vi "MicrometerDryRun.vi"() -> ()   [LabVIEW 2015]
uses:
  <vilib>/Analysis/baseanly.llb/Mean (DBL).vi
  <vilib>/Analysis/NI_AALBase.lvlib
panel:
  in  "Done ?":bool
  out "nome file":string="micrometer_"
  in  "suffisso (se necessario)":string
  out "rms value":dbl format="%0.2f"
  out "mean":dbl format="%0.2f"
  out "appended array":dbl[](array[numeric])
  in  "stop":bool
  in  "2200,500":dbl format="%.2g"
  in  "0,500":dbl format="%.2g"
  in  "0,400":dbl format="%.2g"
  in  "2000,200":dbl format="%.2g"
  in  "1550,200":dbl format="%.2g"
  in  "1200,200":dbl format="%.2g"
  in  "800,200":dbl format="%.2g"
  in  "200,200":dbl format="%.2g"
  in  "2000,1100":dbl format="%.2g"
  in  "1550,1100":dbl format="%.2g"
  in  "1200, 1100":dbl format="%.2g"
  in  "800,1100":dbl format="%.2g"
  in  "200,1100":dbl format="%.2g"
  # "Dry Run"
  # "- Scrivi i valori delle misure effettuate con il micrometro nelle                                  caselle corrispondenti\n- Aggiungi il suffisso al nome del file (se necessario)\n- clicca su \"DONE\" quando hai immesso tutti i valori"
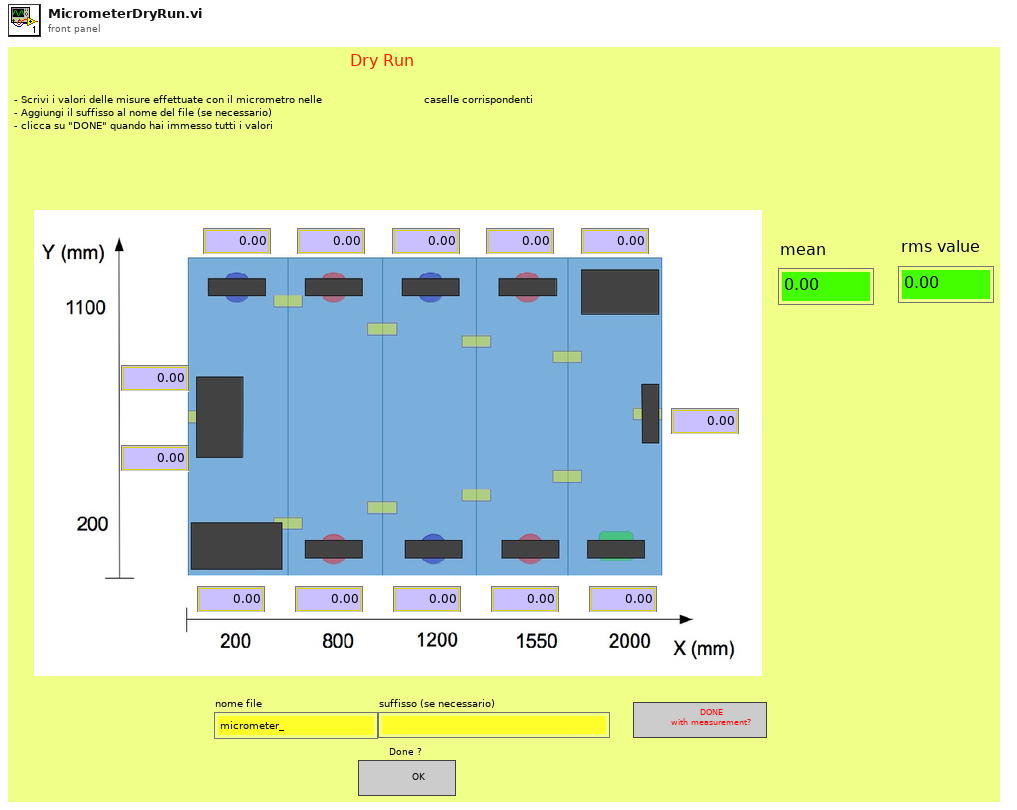
[diagram p1: front panel]
types:
  T1 = enum16{"open", "replace", "create", "open or create", "replace or create", "replace or create with confirmation"}
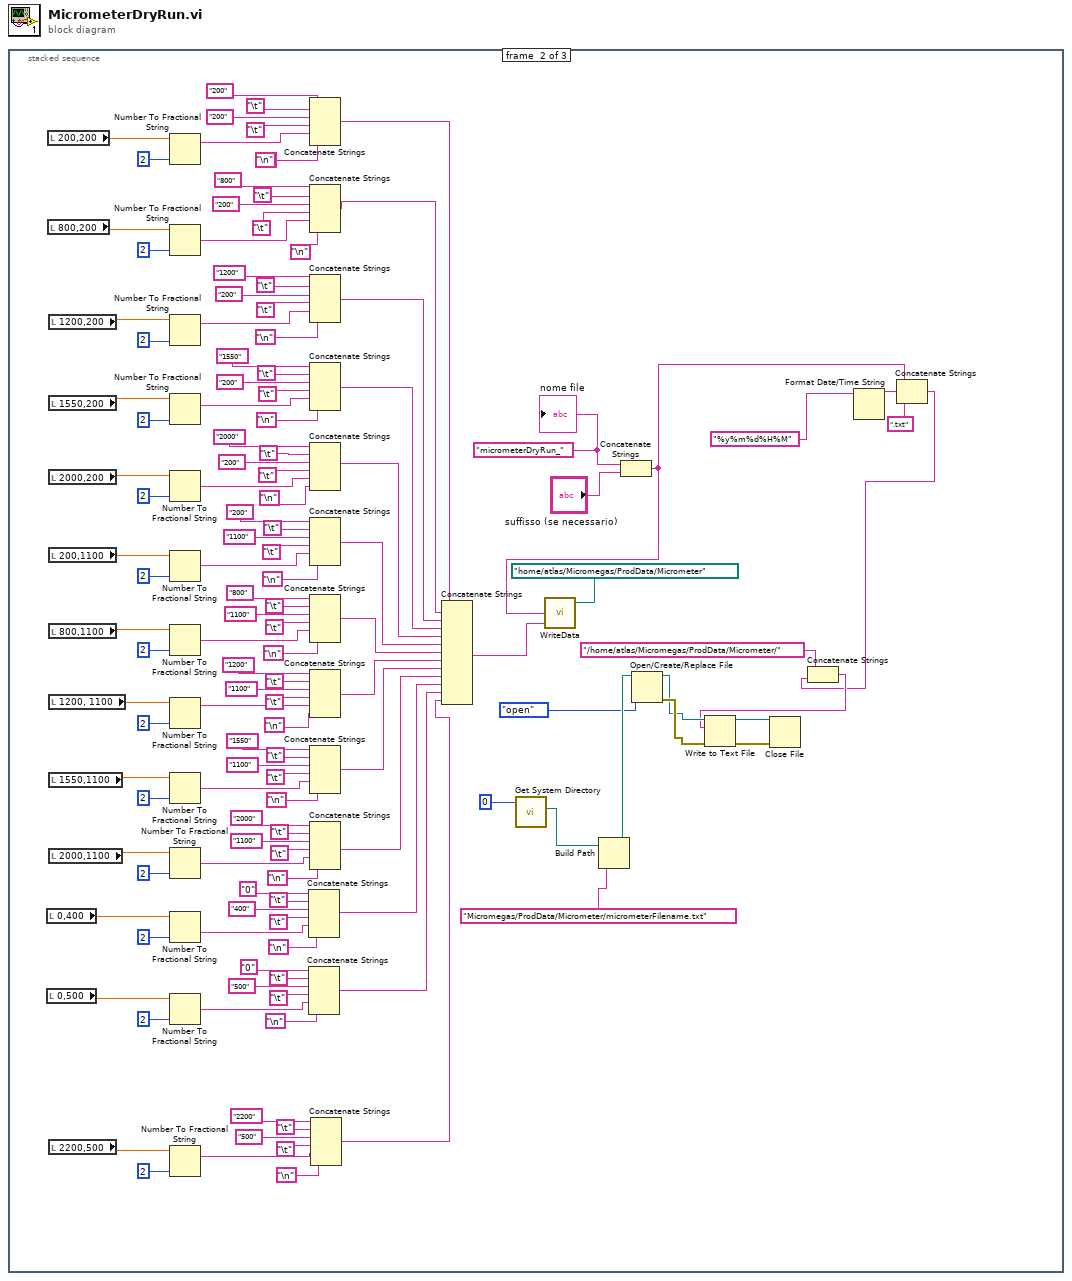
[diagram p0: block diagram]
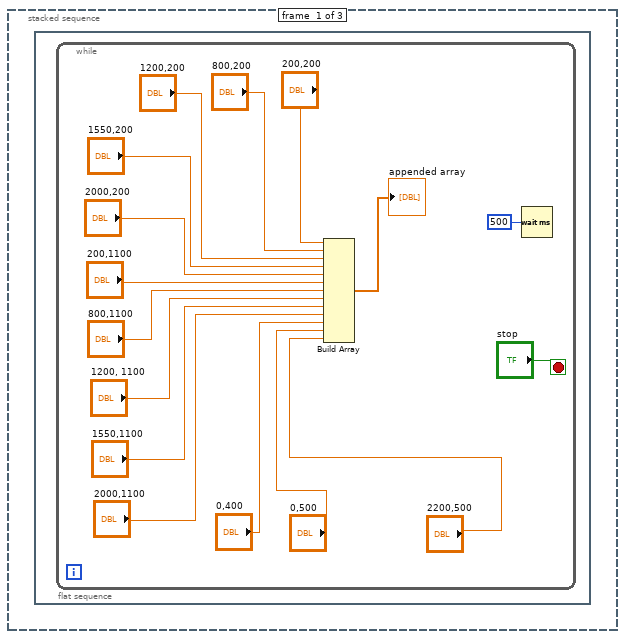
[diagram p2: hidden frame]
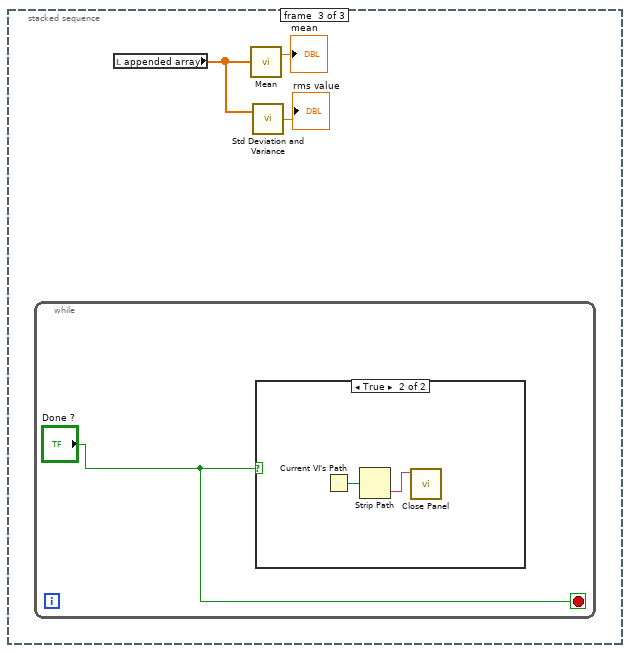
[diagram p3: hidden frame]
diagram:
  n1 = stacked-sequence {
    frame #0 {
      n2 = flat-sequence {
        frame #0 {
          n3 = while {
            stop <- "stop" stop-if-true
            n4 = Build Array("200,200", "800,200", "1200,200", "1550,200", "2000,200", "200,1100", "800,1100", "1200, 1100", "1550,1100", "2000,1100", "0,400", "0,500", "2200,500") -> (→"appended array":dbl[])
            n5 = Wait (ms)(milliseconds to wait=u32 500) -> ()  [unwired: 1 out]
          }
        }
      }
    }
    frame #1 {
      w36 = "micrometerDryRun_" ("string")
      (unwired) "\n"
      n6 = local read "0,400"() -> (w56:dbl)
      n7 = local read "0,500"() -> (w55:dbl)
      n8 = local read "200,200"() -> (w139:dbl)
      n9 = local read "800,200"() -> (w138:dbl)
      n10 = local read "1200,200"() -> (w116:dbl)
      n11 = local read "1550,200"() -> (w115:dbl)
      n12 = local read "2000,200"() -> (w114:dbl)
      n13 = local read "200,1100"() -> (w79:dbl)
      n14 = local read "800,1100"() -> (w78:dbl)
      n15 = local read "1200, 1100"() -> (w77:dbl)
      n16 = local read "1550,1100"() -> (w76:dbl)
      n17 = local read "2000,1100"() -> (w75:dbl)
      n18 = local read "2200,500"() -> (w54:dbl)
      n19 = Number To Fractional String(number=w139, precision (6)=i16 2) -> (F-format string=w148:string)  [unwired: 2 in]
      n20 = Number To Fractional String(number=w138, precision (6)=i16 2) -> (F-format string=w142:string)  [unwired: 2 in]
      n21 = Number To Fractional String(number=w116, precision (6)=i16 2) -> (F-format string=w125:string)  [unwired: 2 in]
      n22 = Number To Fractional String(number=w115, precision (6)=i16 2) -> (F-format string=w131:string)  [unwired: 2 in]
      n23 = Number To Fractional String(number=w114, precision (6)=i16 2) -> (F-format string=w137:string)  [unwired: 2 in]
      n24 = Number To Fractional String(number=w79, precision (6)=i16 2) -> (F-format string=w113:string)  [unwired: 2 in]
      n25 = Number To Fractional String(number=w78, precision (6)=i16 2) -> (F-format string=w106:string)  [unwired: 2 in]
      n26 = Number To Fractional String(number=w77, precision (6)=i16 2) -> (F-format string=w88:string)  [unwired: 2 in]
      n27 = Number To Fractional String(number=w76, precision (6)=i16 2) -> (F-format string=w95:string)  [unwired: 2 in]
      n28 = Number To Fractional String(number=w75, precision (6)=i16 2) -> (F-format string=w85:string)  [unwired: 2 in]
      n29 = Number To Fractional String(number=w56, precision (6)=i16 2) -> (F-format string=w74:string)  [unwired: 2 in]
      n30 = Number To Fractional String(number=w55, precision (6)=i16 2) -> (F-format string=w68:string)  [unwired: 2 in]
      n31 = Number To Fractional String(number=w54, precision (6)=i16 2) -> (F-format string=w62:string)  [unwired: 2 in]
      n32 = Concatenate Strings("0", "\t", "400", "\t", w74, "\n") -> (w39:string)
      n33 = Concatenate Strings("0", "\t", "500", "\t", w68, "\n") -> (w38:string)
      n34 = Concatenate Strings("200", "\t", "200", "\t", w148, "\n") -> (w49:string)
      n35 = Concatenate Strings("800", "\t", "200", "\t", w142, "\n") -> (w48:string)
      n36 = Concatenate Strings("1200", "\t", "200", "\t", w125, "\n") -> (w47:string)
      n37 = Concatenate Strings("1550", "\t", "200", "\t", w131, "\n") -> (w46:string)
      n38 = Concatenate Strings("2000", "\t", "200", "\t", w137, "\n") -> (w45:string)
      n39 = Concatenate Strings("200", "\t", "1100", "\t", w113, "\n") -> (w44:string)
      n40 = Concatenate Strings("800", "\t", "1100", "\t", w106, "\n") -> (w43:string)
      n41 = Concatenate Strings("1200", "\t", "1100", "\t", w88, "\n") -> (w42:string)
      n42 = Concatenate Strings("1550", "\t", "1100", "\t", w95, "\n") -> (w41:string)
      n43 = Concatenate Strings("2000", "\t", "1100", "\t", w85, "\n") -> (w40:string)
      n44 = Concatenate Strings("2200", "\t", "500", "\t", w62, "\n") -> (w33:string)
      n45 = Concatenate Strings(w49, w48, w47, w46, w45, w44, w43, w42, w41, w40, w39, w38, w33) -> (w37:string)
      n46 = call <vilib>:"Get System Directory.vi"("system directory type"=0) -> ("system directory"=w31:path)  [unwired: 10 in]
      n47 = Build Path(base path=w31, name or relative path="Micromegas/ProdData/Micrometer/micrometerFilename.txt") -> (appended path=w32:path)
      n48 = Concatenate Strings(w36, "suffisso (se necessario)") -> (w18:string)
      n49 = call "WriteData.vi"("Message"=w37, "File Prefix"=w18, "base path"=path "/home/atlas/Micromegas/ProdData/Micrometer") -> ()
      n50 = Open/Create/Replace File(file path (use dialog)=w32, operation (0:open)=T1."open") -> (refnum out=w26:refnum<file>, error out=w27:errorcluster)  [unwired: 4 in, 1 out]
      n51 = Format Date/Time String(time format string (%c)="%y%m%d%H%M") -> (date/time string=w21:string)  [unwired: 2 in]
      n52 = Concatenate Strings(w18, w21, ".txt" ("string")) -> (w17:string)
      n53 = Concatenate Strings("/home/atlas/Micromegas/ProdData/Micrometer/", w17) -> (w24:string)
      n54 = Write to Text File(file (use dialog)=w26, text=w24, error in=w27) -> (refnum out=w22:refnum<file>, error out=w23:errorcluster)  [unwired: 1 in, 1 out]
      n55 = Close File(refnum=w22, error in=w23) -> ()  [unwired: 2 out]
      "nome file" <- w36
    }
    frame #2 {
      n56 = while {
        stop <- "Done ?" stop-if-true
        n57 = case shown="True" "Done ?" {
          frame False {
          }
          frame True {
            n58 = Current VI's Path() -> (path=w158:path)
            n59 = Strip Path(path=w158) -> (name=w159:string)  [unwired: 1 out]
            n60 = call <vilib>:"Close Panel.vi"("VI name"=w159) -> ()  [unwired: 10 in, 1 out]
          }
        }
      }
      n61 = local read "appended array"() -> (w155:dbl[])
      n62 = call-poly <vilib>:"Mean.vi"("X"=w155) -> ("mean"=→"mean":dbl)  [unwired: 1 out]
      n63 = call <vilib>:"Std Deviation and Variance.vi"("X"=w155) -> ("standard deviation"=→"rms value":dbl)  [unwired: 1 in, 2 out]
    }
  }
